vi "Unpack Message.vi"(8 "error in (no error)":errorcluster, 9 "Packed Message":string, 10 "Message Name":string, 11 "Message Double in":refnum<class "Message Boolean Array.lvclass">) -> (0 "error out":errorcluster, 2 "Valid":bool, 3 "Message Double out":refnum<class "Message Boolean Array.lvclass">)   [LabVIEW 2016, in "Stream Mediator.lvlib" / "Message Boolean Array.lvclass"]
uses:
  <userlib>/Composed Systems/Stream/Mediator/Classes/Message Boolean Array/Message Boolean Array.lvclass
  C:/Program Files (x86)/National Instruments/LabVIEW 2016/user.lib/Composed Systems/Stream/Mediator/Classes/Message Interface/Message Interface.lvclass
  <userlib>/Composed Systems/Stream/Mediator/Classes/Message Boolean Array/Message Boolean Array.lvclass/Message Boolean Array.ctl
  <userlib>/Composed Systems/Stream/Mediator/Classes/Message Interface/Message Interface.lvclass
  <vilib>/addons/_JKI.lib/Serialization/JSON/JKI JSON Serialization.lvlib
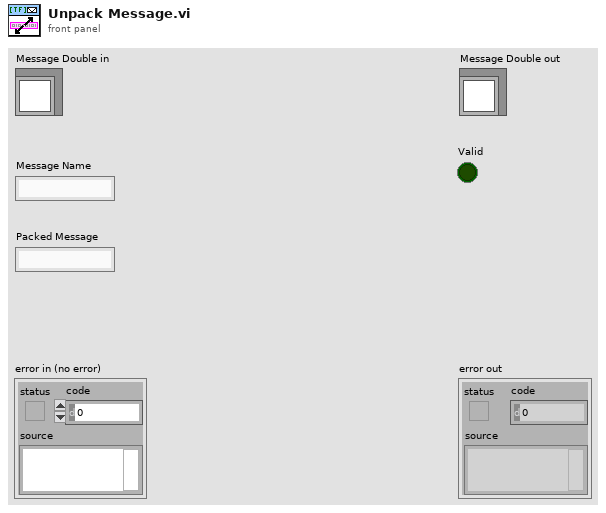
[diagram p1: front panel]
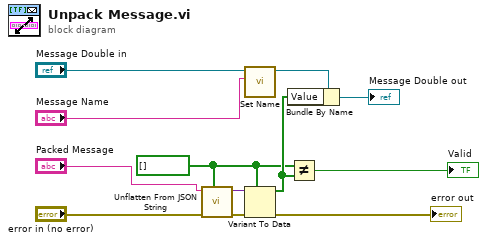
[diagram p0: block diagram]
diagram:
  w2 = bool[] []
  n1 = call <vilib>:"Unflatten From JSON String.vi"("Type and Defaults"=w2, "error in (no error)"="error in (no error)", "JSON String"="Packed Message") -> ("error out"=w6:errorcluster, "Variant"=w8:variant)  [unwired: 7 in]
  n2 = call <userlib>:"Set Name.vi"("Name"="Message Name", "Message Interface in"="Message Double in") -> ("Message Interface out"=w10:refnum<class "Message Boolean Array.lvclass">)  [unwired: 8 in, 1 out]
  n3 = Variant To Data(error in=w6, type=w2, Variant=w8) -> (data=w3:bool[], error out=→"error out":errorcluster)
  n4 = Bundle By Name(cluster=w10, "Value"=w3) -> (→"Message Double out":refnum<class "Message Boolean Array.lvclass">)
  n5 = Not Equal?(x=w2, y=w3) -> (x != y?=→"Valid":bool)
